vi "SetSwerveConfig.vi"   [LabVIEW 2018]
types:
  T1 = enum16{"open", "replace", "create", "open or create", "replace or create", "replace or create with confirmation"}
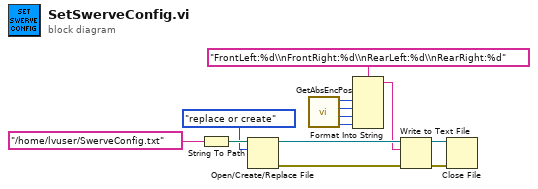
[diagram p0: block diagram]
diagram:
  n1 = String To Path(string="/home/lvuser/SwerveConfig.txt" ("directory path")) -> (path=w11:path)
  n2 = Open/Create/Replace File(file path (use dialog)=w11, operation (0:open)=T1."replace or create") -> (refnum out=w9:refnum<file>, error out=w8:errorcluster)  [unwired: 4 in, 1 out]
  n3 = call "GetAbsEncPos.vi"() -> ("RearRightPulsePos"=w2:i32, "RearLeftPulsePos"=w3:i32, "FrontRightPulsePos"=w4:i32, "FrontLeftPulsePos"=w5:i32)  [unwired: 8 in]
  n4 = Format Into String(format string="FrontLeft:%d\\nFrontRight:%d\\nRearLeft:%d\\nRearRight:%d", w5, w4, w3, w2) -> (resulting string=w1:string)  [unwired: 2 in, 1 out]
  n5 = Write to Text File(file (use dialog)=w9, text=w1, error in=w8) -> (refnum out=w12:refnum<file>, error out=w7:errorcluster)  [unwired: 1 in, 1 out]
  n6 = Close File(refnum=w12, error in=w7) -> ()  [unwired: 2 out]
